vi "bmp_2_mat.vi"(9 "Destinatia1":path, 11 "Imaginea1":path) -> ()   [LabVIEW 2015]
uses:
  <vilib>/picture/picture.llb/Draw True-Color Pixmap.vi
panel:
  out "new":u8[][](array[numeric]) format="%x"
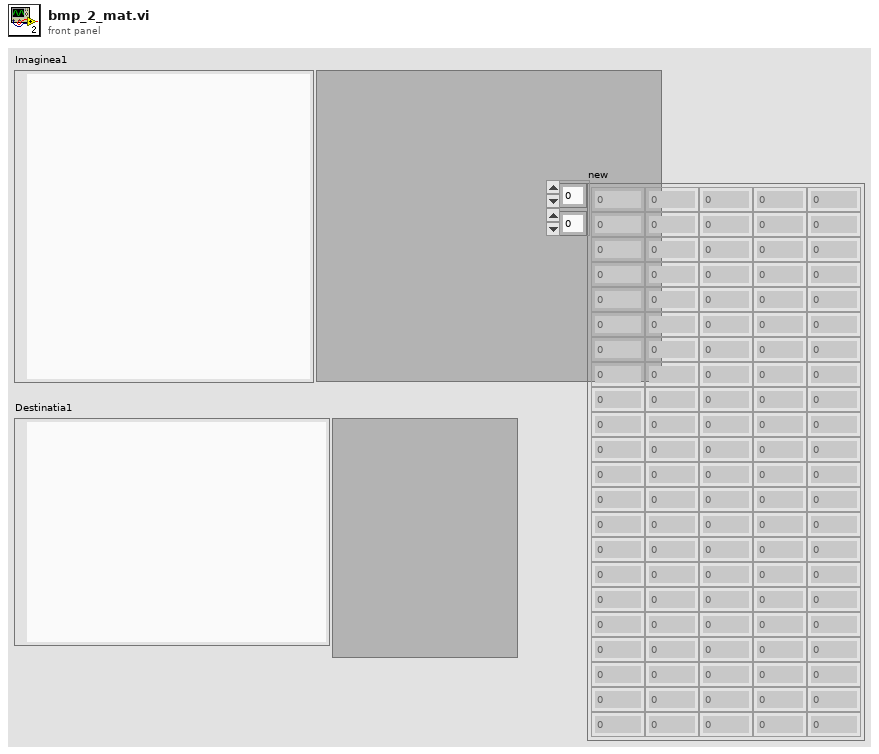
[diagram p1: front panel]
types:
  T1 = typedef "imagedata.ctl" = cluster{"image type":i32, "image depth":i32, "image":u8[], "mask":u8[], "colors":u32[], "Rectangle":cluster{"left":i16, "top":i16, "right":i16, "bottom":i16}}
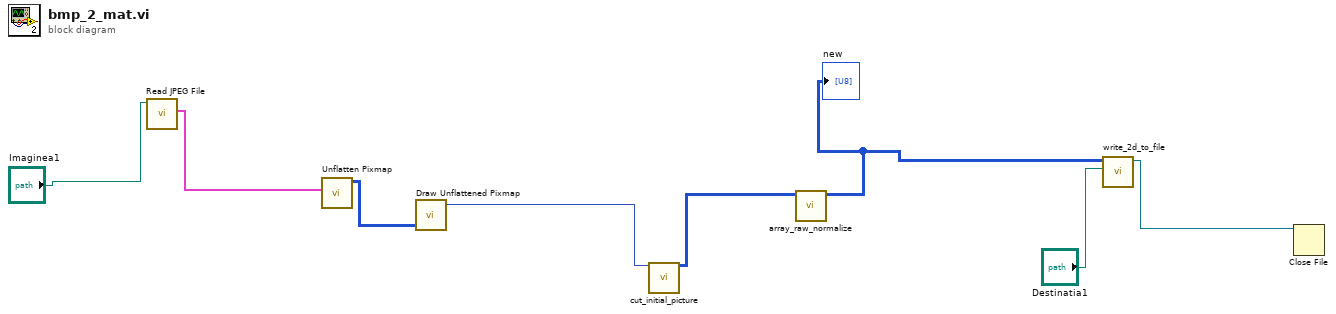
[diagram p0: block diagram]
diagram:
  n1 = call <vilib>:"Read JPEG File.vi"("path to JPEG file"="Imaginea1") -> ("image data"=w2:T1)  [unwired: 8 in, 2 out]
  n2 = call <vilib>:"Unflatten Pixmap.vi"("image data"=w2) -> ("24-bit pixmap"=w4:u32[][])  [unwired: 4 in, 6 out]
  n3 = call-poly <vilib>:"Draw Unflattened Pixmap.vi"("data (RGB format)"=w4) -> ("new picture"=w5:picture)  [unwired: 8 in]
  n4 = call "cut_initial_picture.vi"("picture"=w5) -> ("new"=w1:u32[][])  [unwired: 14 in]
  n5 = call "array_raw_normalize.vi"("array"=w1) -> ("Array"=w8:u8[][])  [unwired: 10 in]
  "new" <- w8
  n6 = call "write_2d_to_file.vi"("Path 2"="Destinatia1", "Array"=w8) -> ("refnum out"=w7:refnum<file>)  [unwired: 9 in]
  n7 = Close File(refnum=w7) -> ()  [unwired: 1 in, 2 out]
